vi "Progress_Local_For_Loop-1.vi"(1 "[IN] Number of Frames":i32, 2 "[IN] Current Index":i32) -> (0 "[OUT] % progress":u8)   [LabVIEW 2017]
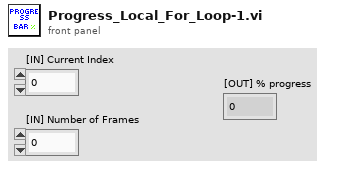
[diagram p1: front panel]
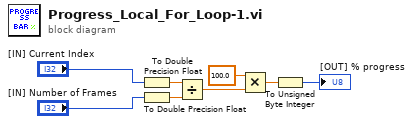
[diagram p0: block diagram]
diagram:
  n1 = To Double Precision Float(number="[IN] Current Index") -> (double precision float=w7:dbl)
  n2 = To Double Precision Float(number="[IN] Number of Frames") -> (double precision float=w5:dbl)
  n3 = Divide(x=w7, y=w5) -> (x/y=w4:dbl)
  n4 = Multiply(x=100.0, y=w4) -> (x*y=w2:dbl)
  n5 = To Unsigned Byte Integer(number=w2) -> (unsigned 8bit integer=→"[OUT] % progress":u8)
